vi "Write Strings [].vi"(8 "error in (no error)":errorcluster, 10 "Strings []":string[](array[string]), 11 "MixedCheckbox.lvclass in":refnum<class "MixedCheckbox.lvclass">) -> (0 "error out":errorcluster, 3 "MixedCheckbox.lvclass out":refnum<class "MixedCheckbox.lvclass">)   [LabVIEW 2015, in "MixedCheckbox.lvclass"]
uses:
  MixedCheckbox.lvclass
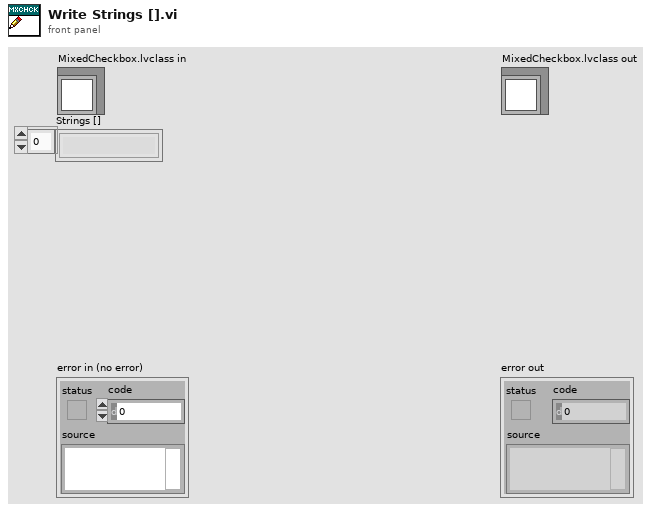
[diagram p1: front panel]
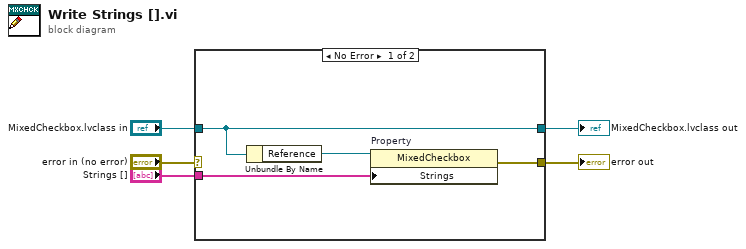
[diagram p0: block diagram]
diagram:
  n1 = case shown="No Error" "error in (no error)" {
    selector: "error in (no error)" -> [_ w11]
    tunnel: [w9 w11] -> w4
    tunnel: [w7 w10] -> w2
    tunnel: "MixedCheckbox.lvclass in" -> [w7 w10]
    tunnel: "Strings []" -> [w8 _]
    frame No Error {
      n2 = Unbundle By Name(w7) -> ("Reference"=w6:refnum<vi>)
      n3 = property on="Property" class="MixedCheckbox"(reference=w6, "Strings"=w8) -> (error out=w9:errorcluster)  [unwired: 1 in, 1 out]
    }
    frame Error {
    }
  }
  "error out" <- w4
  "MixedCheckbox.lvclass out" <- w2
